vi "sensor de humedad 2.vi"(6 "Error In":errorcluster, 8 "Pin S. Humedad":u8, 9 "LINX Resource":T2) -> (0 "Error Out":errorcluster, 1 "Porcentaje de humedad":string, 2 "Nivel de Humedad.":T1, 4 "LINX Resource 2":T2, 5 "Nivel de humedad":string)   [LabVIEW 2013]
uses:
  <vilib>/MakerHub/LINX/Private/Type Defs/LINX Ref.ctl
  <vilib>/MakerHub/LINX/Private/Type Defs/Platform.ctl
  <vilib>/MakerHub/LINX/Private/Type Defs/Interface.ctl
  <vilib>/MakerHub/LINX/Private/Device/Type Defs/LINX Device Config.ctl
  <vilib>/MakerHub/LINX/Private/Device/Type Defs/TCP Config.ctl
  <vilib>/MakerHub/LINX/Private/Device/Type Defs/Channels.ctl
  <vilib>/MakerHub/LINX/Public/Peripherals/Analog/Analog Read 1 Chan.vi
  <vilib>/MakerHub/LINX/LMH-LINX.lvlib
  <vilib>/MakerHub/LINX/Private/Device/Device.lvlib
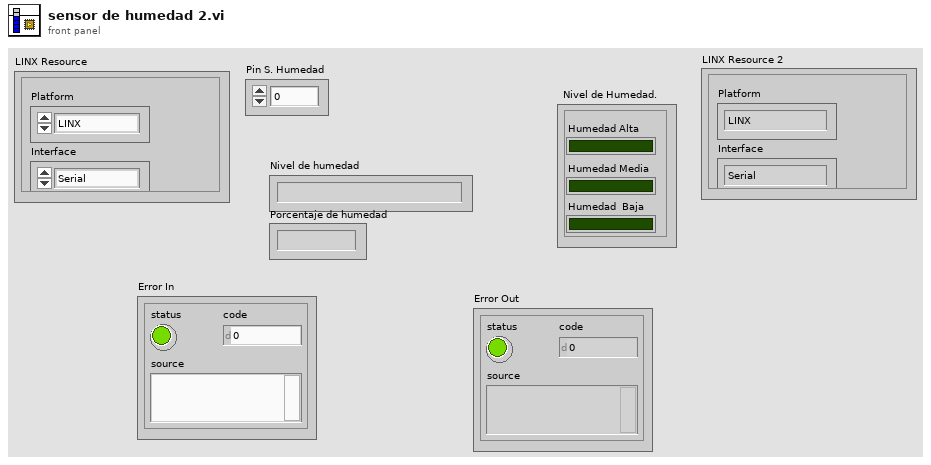
[diagram p1: front panel]
types:
  T1 = cluster{"Humedad Alta":bool, "Humedad  Baja":bool, "Humedad Media":bool}
  T2 = typedef "LMH-LINX.lvlib/LINX Ref.ctl" = cluster{"Platform":T3, "Interface":T4, "LINX Device Config":T5}
  T3 = typedef "LMH-LINX.lvlib/Platform.ctl" = enum16{"LINX", "myRIO"}
  T4 = typedef "LMH-LINX.lvlib/Interface.ctl" = enum16{"Serial", "TCP"}
  T5 = typedef "LMH-LINX.lvlib/Device.lvlib/LINX Device Config.ctl" = cluster{"Interface":T4, "COM Port":refnum<visa-resource-name>, "TCP Configuration":T6, "Device Family":u8, "Device ID":u8, "Device Name":string, "TCP Ref":refnum<k5>, "Channels":T7}
  T6 = typedef "LMH-LINX.lvlib/Device.lvlib/TCP Config.ctl" = cluster{"IP Address":string, "Port":u16}
  T7 = typedef "LMH-LINX.lvlib/Channels.ctl" = cluster{"DI":u8[], "DO":u8[], "AI":u8[], "AO":u8[], "PWM":u8[], "QE":u8[], "UART":u8[], "I2C 2":u8[], "SPI":u8[], "CAN":u8[], "Servo":u8[], "AI Ref (V)":dbl, "AO Ref (V)":dbl, "AO Resolution (Bits)":u8}
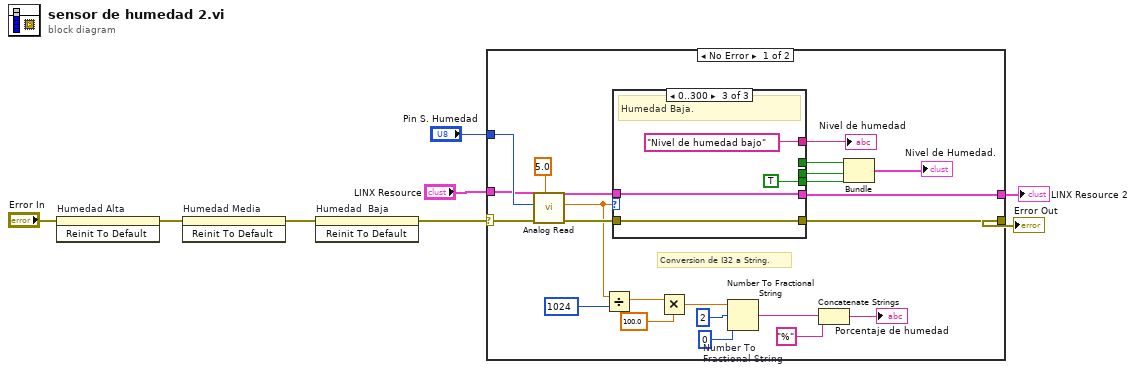
[diagram p0: block diagram]
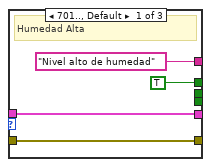
[diagram p2: hidden frame]
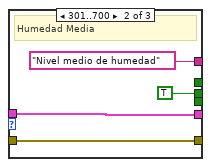
[diagram p3: hidden frame]
diagram:
  n1 = invoke on="Humedad Alta" class="Bool (strict)" method="Reinit To Default"(error in="Error In") -> (error out=w8:errorcluster)  [unwired: 2 in, 2 out]
  n2 = invoke on="Humedad Media" class="Bool (strict)" method="Reinit To Default"(error in=w8) -> (error out=w7:errorcluster)  [unwired: 2 in, 2 out]
  n3 = invoke on="Humedad  Baja" class="Bool (strict)" method="Reinit To Default"(error in=w7) -> (error out=w4:errorcluster)  [unwired: 2 in, 2 out]
  n4 = case shown="No Error" w4 {
    selector: w4 -> [w20 w45]
    tunnel: [w21 w45] -> w1
    tunnel: [w17 w44] -> w2
    tunnel: "Pin S. Humedad" -> [w16 _]
    tunnel: "LINX Resource" -> [w13 w44]
    frame No Error {
      # "Conversion de I32 a String."
      n5 = call-poly <vilib>:"Analog Read.vi"("AI Range (V)"=5.0, "Error In"=w20, "Analog Channel"=w16, "LINX Resource"=w13) -> ("Error Out"=w19:errorcluster, "AI Value"=w14:dbl, "LINX Resource"=w18:T2)  [unwired: 4 in, 1 out]
      n6 = Divide(x=w14, y=i16 1024) -> (x/y=w30:dbl)
      n7 = case shown="0..300" w14 {
        tunnel: ["Nivel alto de humedad" "Nivel medio de humedad" "Nivel de humedad bajo"] -> w24
        tunnel: w19 -> [w34 w38 w42]
        tunnel: [w34 w38 w42] -> w21
        tunnel: w18 -> [w33 w37 w41]
        tunnel: [w33 w37 w41] -> w17
        tunnel: [TRUE _ _] -> w12
        tunnel: [_ TRUE _] -> w11
        tunnel: [_ _ TRUE] -> w10
        frame 701.., Default {
          # "Humedad Alta"
        }
        frame 301..700 {
          # "Humedad Media"
        }
        frame 0..300 {
          # "Humedad Baja."
        }
      }
      "Nivel de humedad" <- w24
      n8 = Multiply(x=w30, y=100.0) -> (x*y=w28:dbl)
      n9 = Number To Fractional String "Number To \nFractional String"(number=w28, width (-)=i16 2, precision (6)=i16 0) -> (F-format string=w23:string)  [unwired: 1 in]
      n10 = Concatenate Strings(w23, "%") -> (→"Porcentaje de humedad":string)
      n11 = Bundle(w12, w11, w10) -> (→"Nivel de Humedad.":cluster{bool, bool, bool})  [unwired: 1 in]
    }
    frame Error {
    }
  }
  "Error Out" <- w1
  "LINX Resource 2" <- w2
